vi "OP300ZP_SCANequipements.vi"(8 "Errin":errorcluster caption="errin", 10 "Chaîne":string="Log et conf\\Config.ini", 11 "pathin":path=path "D:/CODE/02 SLIM ZEN") -> (0 "errout 2":errorcluster={"status"=TRUE, "code"=0, "source"="PCAN_CHANNEL ILLEGAL"} caption="errout", 1 "KO?":bool=TRUE, 3 "VISA OUT":T1)   [LabVIEW 2020]
doc: "Ce vi il détecte la presence des équipements"
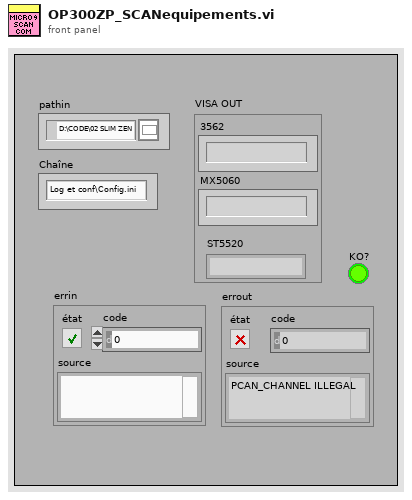
[diagram p1: front panel]
types:
  T1 = cluster{"3562":string, "MX5060":string, "ST5520":string}
  T2 = cluster{"3562":string, "MX5060":string, "ST5520":string, "ATEQ":string}
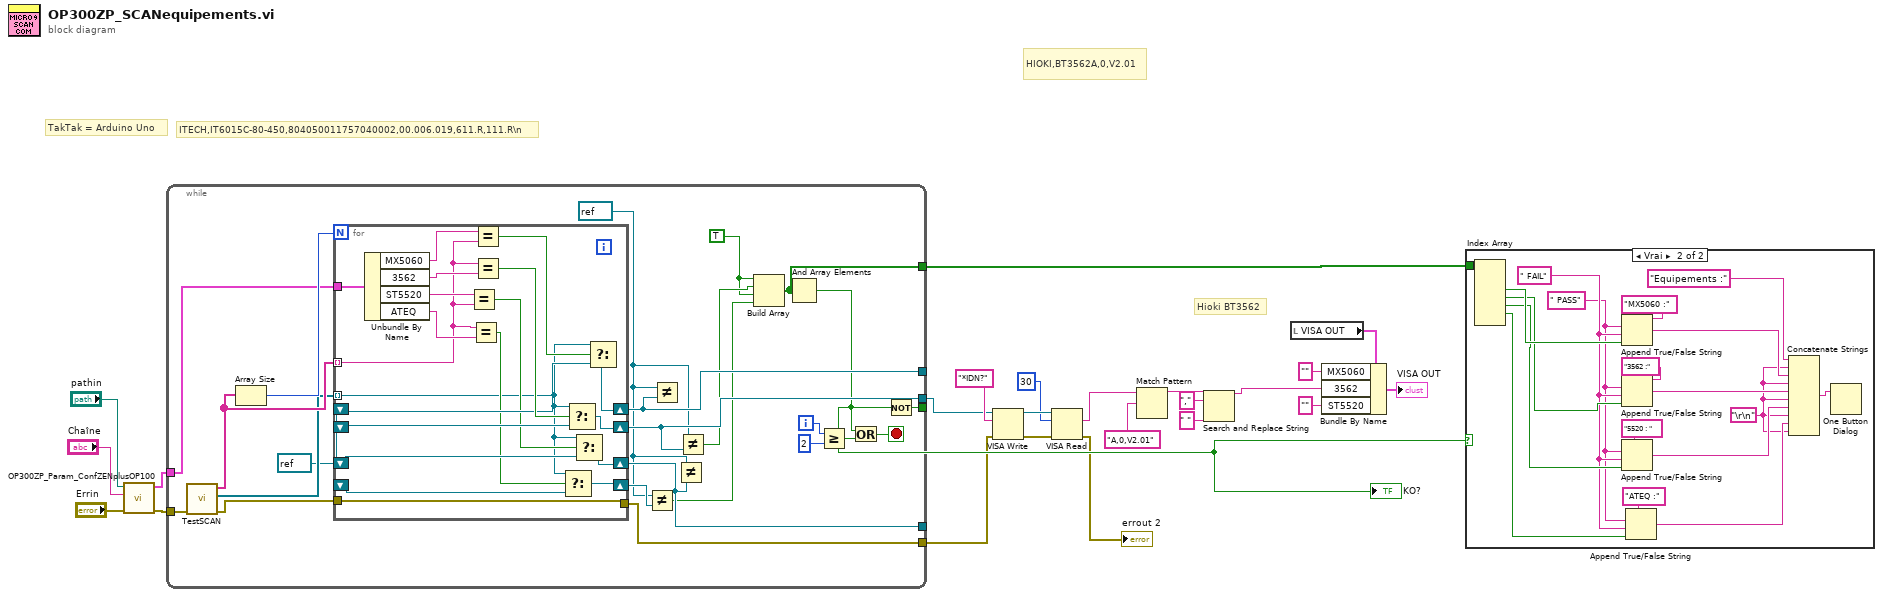
[diagram p0: block diagram]
diagram:
  # "HIOKI,BT3562A,0,V2.01"
  # "Hioki BT3562"
  # "TakTak = Arduino Uno"
  # "ITECH,IT6015C-80-450,804050011757040002,00.006.019,611.R,111.R\\n"
  n1 = call "OP300ZP_Param_ConfZENplusOP100.vi"("errin"="Errin", "Chaîne"="Chaîne", "pathin"="pathin") -> ("errout"=w21:errorcluster, "VISA OUT"=w20:T2)  [unwired: 7 in]
  n2 = while {
    tunnel: [w37] -> _
    tunnel: [w36] -> w16
    tunnel: w21 -> [w46]
    tunnel: [w41] -> w24
    tunnel: w20 -> [w38]
    tunnel: [w34] -> w23
    tunnel: [w32] -> _
    tunnel: [w28] -> w13
    i -> [w40]
    stop <- w43 stop-if-true
    w29 = TRUE ("élément")
    w26 = refnum<visa-resource-name> refnum ("x")
    w33 = refnum<visa-resource-name> refnum ("VISA resource name out")
    n3 = call "TestSCAN.vi"("errin"=w46) -> ("error out"=w31:errorcluster, "Tableau 2"=w44:refnum<visa-resource-name>[], "Tableau"=w45:string[])  [unwired: 8 in]
    n4 = Array Size(array=w45) -> (size(s)=w47:i32)
    n5 = for {
      N: w47 -> [_]
      shift-right: [w65] -> w37
      shift-left: w33 -> [w63]
      shift-right: [w64] -> w36
      shift-left: w33 -> [w62]
      tunnel: w45 -> [w52] mode=indexing
      tunnel: w38 -> [w61]
      shift-right: [w58] -> w32
      shift-left: w33 -> [w59]
      tunnel: w44 -> [w50] mode=indexing
      tunnel: w31 -> [w54]
      tunnel: [w54] -> w28
      shift-right: [w48] -> w27
      shift-left: _ -> [w49]
      n6 = Unbundle By Name(w61) -> ("MX5060"=w60:string, "3562"=w55:string, "ST5520"=w57:string, "ATEQ"=w53:string)
      n7 = Equal?(x=w57, y=w52) -> (x = y?=w56:bool)
      n8 = Equal?(x=w52, y=w53) -> (x = y?=w51:bool)
      n9 = Equal?(x=w60, y=w52) -> (x = y?=w66:bool)
      n10 = Equal?(x=w52, y=w55) -> (x = y?=w67:bool)
      n11 = Select(t=w50, s=w51, f=w49) -> (s? t:f=w48:refnum<visa-resource-name>)
      n12 = Select(t=w50, s=w67, f=w62) -> (s? t:f=w64:refnum<visa-resource-name>)
      n13 = Select(t=w50, s=w56, f=w59) -> (s? t:f=w58:refnum<visa-resource-name>)
      n14 = Select(t=w50, s=w66, f=w63) -> (s? t:f=w65:refnum<visa-resource-name>)
    }
    n15 = Not Equal?(x=w26, y=w27) -> (x != y?=w25:bool)
    n16 = Not Equal?(x=w26, y=w37) -> ()  [unwired: 1 out]
    n17 = Not Equal?(x=w32, y=w26) -> ()  [unwired: 1 out]
    n18 = Not Equal?(x=w26, y=w36) -> (x != y?=w30:bool)
    n19 = Build Array(w29, w30, w29, w25) -> (w34:bool[])
    n20 = And Array Elements(Boolean array=w34) -> (logical AND=w35:bool)
    n21 = Greater Or Equal?(x=w40, y=2) -> (x >= y?=w42:bool)
    n22 = Or(x=w35, y=w42) -> (x .or. y?=w43:bool)
    n23 = Not(x=w35) -> (.not. x?=w41:bool)
  }
  "KO?" <- w24
  n24 = VISA Write(VISA resource name=w16, write buffer="*IDN?" ("buffer d'écriture"), error in (no error)=w13) -> (VISA resource name out=w15:refnum<visa-resource-name>, error out=w12:errorcluster)  [unwired: 1 out]
  n25 = VISA Read(VISA resource name=w15, byte count=u32 30 ("nombre d'octets"), error in (no error)=w12) -> (read buffer=w10:string, error out=→"errout 2":errorcluster)  [unwired: 2 out]
  n26 = Match Pattern(string=w10, regular expression="A,0,V2.01" ("expression régulière")) -> (before substring=w8:string)  [unwired: 1 in, 3 out]
  n27 = Search and Replace String(input string=w8, search string="," ("chaîne recherchée"), replace string=" " ("chaîne de remplacement (\"\")")) -> (result string=w3:string)  [unwired: 5 in, 3 out]
  n28 = local read "VISA OUT"() -> (w4:T1)
  n29 = Bundle By Name(cluster=w4, "MX5060"="", "3562"=w3, "ST5520"="") -> (→"VISA OUT":T1)
  n30 = case shown="Vrai" w24 {
    tunnel: w23 -> [_ w77]
    frame False {
    }
    frame True {
      w68 = "\r\n"
      w71 = " PASS" ("chaîne faux")
      w72 = " FAIL" ("chaîne faux")
      n31 = Index Array(array=w77) -> (element #2=w76:bool, element #3=w75:bool, element #4=w74:bool, element #5=w70:bool)  [unwired: 6 in, 2 out]
      n32 = Append True/False String(1:w76, 2:w72, 3:w71, 4:"MX5060 :" ("chaîne (\"\")")) -> (0:w81:string)
      n33 = Append True/False String(1:w75, 2:w72, 3:w71, 4:"3562 :" ("chaîne (\"\")")) -> (0:w80:string)
      n34 = Append True/False String(1:w74, 2:w72, 3:w71, 4:"5520 : " ("chaîne (\"\")")) -> (0:w79:string)
      n35 = Append True/False String(1:w70, 2:w72, 3:w71, 4:"ATEQ :" ("chaîne (\"\")")) -> (0:w69:string)
      n36 = Concatenate Strings("Equipements :" ("chaîne"), w68, w81, w68, w80, w68, w79, w68, w69, w68) -> (w78:string)
      n37 = One Button Dialog(message=w78) -> ()  [unwired: 1 in, 1 out]
    }
  }
